vi "Error Query.vi"(8 "error in (no error)":errorcluster, 11 "VISA resource name":refnum<visa-resource-name>) -> (0 "error out":errorcluster, 2 "Error Message":string, 3 "VISA resource name out":refnum<visa-resource-name>)   [LabVIEW 2025, in "Lake Shore 336.lvlib"]
doc: "Queries the instrument for any errors or warnings in the instrument's status system.\n\nThe following conditions will be returned as errors in the Error Out cluster:\n<B>Processor Communication Error</B>\n<B>Query Error</B>\n<B>Execution Error</B>\n<B>Command Error</B>\n<B>Calibration Error</B>\n\nThe following conditions will be returned as warnings in the Error Out cluster:\n<B>Sensor Alarming</B>\n<B>Invalid Reading</B>\n<B>Temperature Underrange</B>\n<B>Temperature Overrange</B>\n<B>Sensor Units Zero</B>\n<B>Sensor Units Overrange</B>\n\nNote:\nThis VI is called automatically by most driver VIs so it is not usually necessary to call this in an application."
uses:
  Lake Shore 336.lvlib
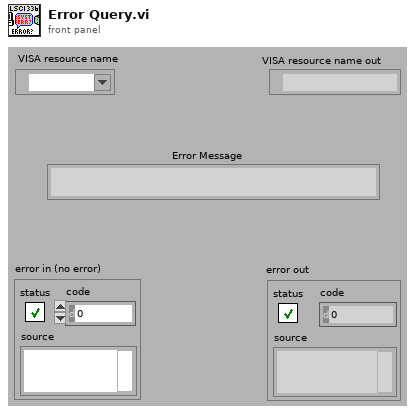
[diagram p1: front panel]
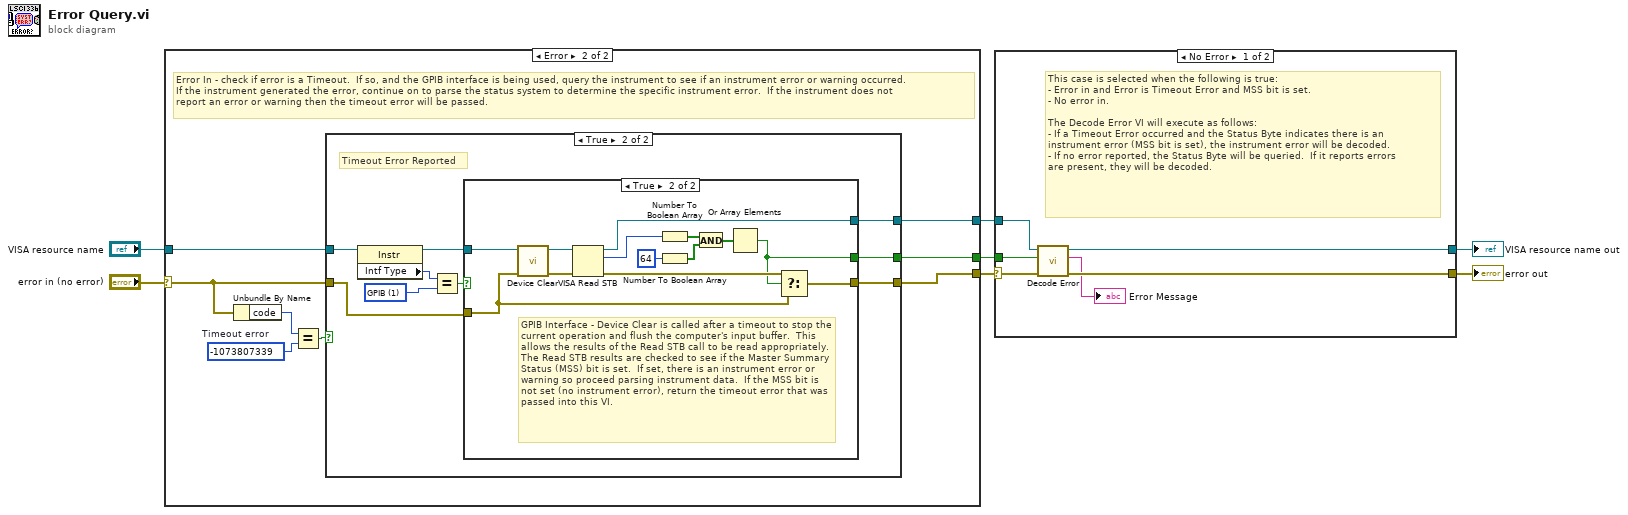
[diagram p0: block diagram]
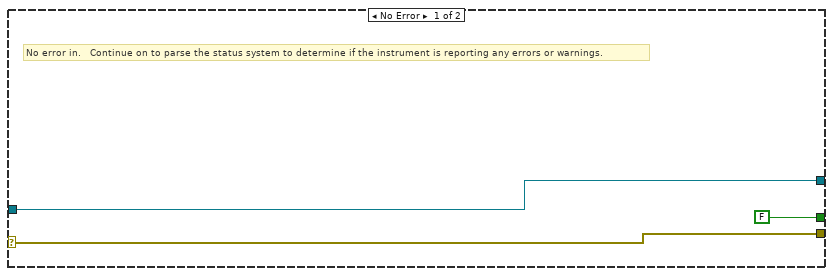
[diagram p2: hidden frame]
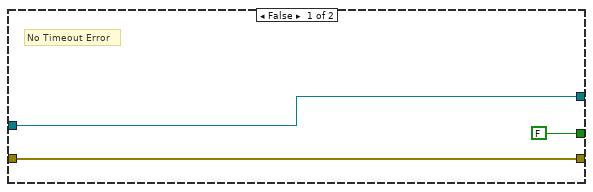
[diagram p3: hidden frame]
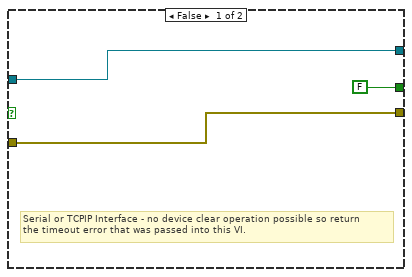
[diagram p4: hidden frame]
diagram:
  n1 = case shown="Error" "error in (no error)" {
    selector: "error in (no error)" -> [w10 w15]
    tunnel: "VISA resource name" -> [w9 w11]
    tunnel: [w10 w14] -> w4
    tunnel: [w9 w13] -> w3
    tunnel: [FALSE w12] -> w2
    frame No Error {
      # "No error in.   Continue on to parse the status system to determine if the instrument is reporting any errors or warnings."
    }
    frame Error {
      w17 = -1073807339  # Timeout error
      # "Error In - check if error is a Timeout.  If so, and the GPIB interface is being used, query the instrument to see if an instrument error or warning occurred.  \nIf the instrument generated the error, continue on to parse the status system to determine the specific instrument error.  If the instrument does not \nreport an error or warning then the timeout error will be passed."
      n2 = Unbundle By Name(w15) -> ("code"=w18:i32)
      n3 = Equal?(x=w18, y=w17) -> (x = y?=w16:bool)
      n4 = case shown="True" w16 {
        tunnel: w15 -> [w21 w23]
        tunnel: [w21 w28] -> w14
        tunnel: [w19 w27] -> w13
        tunnel: [FALSE w26] -> w12
        tunnel: w11 -> [w19 w24]
        frame False {
          # "No Timeout Error"
        }
        frame True {
          w30 = u16 1 items=["GPIB"=1, "VXI"=2, "GPIB-VXI"=3, "Serial"=4, "PXI"=5, "TCPIP"=6, "USB"=7] ("Interface Information:Interface Type")
          # "Timeout Error Reported"
          n5 = property class="Instr"(reference=w24) -> (reference out=w25:refnum<visa-resource-name>, "Intf Type"=w22:u16)  [unwired: 1 in, 1 out]
          n6 = Equal?(x=w22, y=w30) -> (x = y?=w29:bool)
          n7 = case shown="True" w29 {
            tunnel: w23 -> [w31 w36]
            tunnel: [w31 w37] -> w28
            tunnel: w25 -> [w32 w41]
            tunnel: [w32 w38] -> w27
            tunnel: [FALSE w35] -> w26
            frame False {
              # "Serial or TCPIP Interface - no device clear operation possible so return \nthe timeout error that was passed into this VI."
            }
            frame True {
              # "GPIB Interface - Device Clear is called after a timeout to stop the current operation and flush the computer's input buffer.  This allows the results of the Read STB call to be read appropriately.  The Read STB results are checked to see if the Master Summary Status (MSS) bit is set.  If set, there is an instrument error or warning so proceed parsing instrument data.  If the MSS bit is not set (no instrument error), return the timeout error that was passed into this VI."
              n8 = call "Device Clear.vi"("error in (no error)"=w36, "VISA Resource Name"=w41) -> ("error out"=w40:errorcluster, "VISA Resource Out"=w39:refnum<visa-resource-name>)  [unwired: 8 in]
              n9 = VISA Read STB(8:w40, 11:w39) -> (0:w42:errorcluster, 2:w34:u16, 3:w38:refnum<visa-resource-name>)
              n10 = Number To Boolean Array(number=w34) -> (Boolean array=w43:bool[])
              n11 = Number To Boolean Array(number=64) -> (Boolean array=w45:bool[])
              n12 = And(x=w43, y=w45) -> (x .and. y?=w44:bool[])
              n13 = Or Array Elements(Boolean array=w44) -> (logical OR=w35:bool)
              n14 = Select(t=w42, s=w35, f=w36) -> (s? t:f=w37:errorcluster)
            }
          }
        }
      }
    }
  }
  n15 = case shown="No Error" w4 {
    selector: w4 -> [w51 w54]
    tunnel: w3 -> [w52 w53]
    tunnel: w2 -> [w47 _]
    tunnel: [w49 w54] -> w5
    tunnel: [w50 w53] -> w6
    frame No Error {
      # "This case is selected when the following is true:\n- Error in and Error is Timeout Error and MSS bit is set.\n- No error in.\n\nThe Decode Error VI will execute as follows:\n- If a Timeout Error occurred and the Status Byte indicates there is an \ninstrument error (MSS bit is set), the instrument error will be decoded.\n- If no error reported, the Status Byte will be queried.  If it reports errors\nare present, they will be decoded."
      n16 = call "Decode Error.vi"("error in (no error)"=w51, "MSS Bit Set (F: No)"=w47, "VISA resource name"=w52) -> ("error out"=w49:errorcluster, "Error Message"=→"Error Message":string, "VISA resource name out"=w50:refnum<visa-resource-name>)  [unwired: 6 in]
    }
    frame Error {
      # "This case is selected when either of the following is true:\n- Error in and error is Timeout Error AND MSS bit is not set.\n- Error in and error is not a Timeout Error.\n\nThe error will be passed without checking the instrument\nfor additional errors or warnings."
    }
  }
  "error out" <- w5
  "VISA resource name out" <- w6
